vi "LoadFiles.vi"   [LabVIEW 2014]
uses:
  Robot Global Data.vi
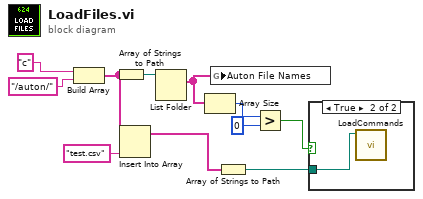
[diagram p0: block diagram]
diagram:
  n1 = Build Array("c", "/auton/") -> (w8:string[])
  n2 = Array of Strings to Path(0:w8) -> (2:w9:path)  [unwired: 1 in]
  n3 = Insert Into Array(array=w8, new element="test.csv" ("new element/subarray")) -> (w7:string[])  [unwired: 1 in]
  n4 = List Folder(path=w9) -> (filenames=w5:string[])  [unwired: 3 in, 3 out]
  n5 = Array Size(array=w5) -> (size(s)=w4:i32)
  n6 = global write "Robot Global Data.vi" "Auton File Names"(w5) -> ()
  n7 = Array of Strings to Path(0:w7) -> (2:w2:path)  [unwired: 1 in]
  n8 = Greater?(x=w4, y=0) -> (0:w1:bool)
  n9 = case shown="True" w1 {
    tunnel: w2 -> [_ w12]
    frame False {
    }
    frame True {
      n10 = call "LoadCommands.vi"("File"=w12) -> ()  [unwired: 11 in]
    }
  }
